vi "climb mode.vi"(4 "i":i32=1508, 6 "Joystick 2":T1, 7 "Arm Angle":dbl=0.38043151000000003, 8 "engage climb":bool, 9 "Button 1":bool, 10 "Slide":dbl(slide)=1.0 scale=0.0..1.0, 11 "Joystick 1 Axes":T2={"Axis 1 (x)"=0.047244094488188976, "Axis 2 (y)"=-0.047244094488188976, "Axis 3 (throttle)"=-1.0, "Axis 4"=0.0, "Axis 5"=0.0, "Axis 6"=0.0}) -> ()   [LabVIEW 2012]
uses:
  <vilib>/Rock Robotics/WPI/Solenoid/WPI_SolenoidValue.ctl
  <vilib>/Rock Robotics/WPI/Joystick/WPI_JoystickGetSetRefNum.vi
  <vilib>/Rock Robotics/WPI/Solenoid/WPI_SolenoidSetEnum.vi
panel:
  out "Arm Motor Output":dbl
  out "Down Range":dbl=0.6
  out "Up Range":dbl=4.1
  out "right f":i32=11868
  out "left f":i32=11868
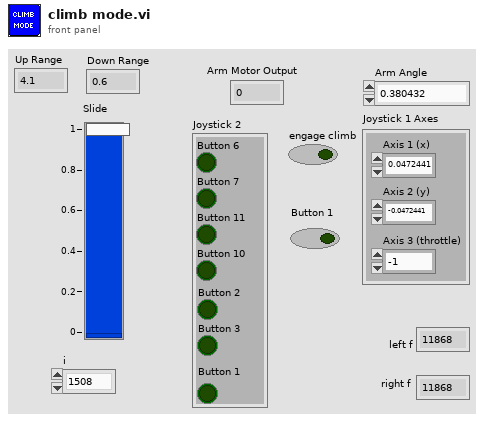
[diagram p1: front panel]
types:
  T1 = cluster{"Button 6":bool, "Button 7":bool, "Button 11":bool, "Button 10":bool, "Button 2":bool, "Button 3":bool, "Button 1":bool}
  T2 = cluster{"Axis 1 (x)":dbl, "Axis 2 (y)":dbl, "Axis 3 (throttle)":dbl, "Axis 4":dbl, "Axis 5":dbl, "Axis 6":dbl}
  T3 = typedef "WPI_SolenoidValue.ctl" = enum16{"Off", "On", "Forward", "Reverse"}
  T4 = typedef "WPI_JoystickDevRef.ctl" = cluster{"Device":T5}
  T5 = typedef "WPI_JoystickDeviceEnum.ctl" = enum16{"USB 1", "USB 2", "USB 3", "USB 4", "Kinect 1", "Kinect 2"}
  T6 = typedef "WPI_JoystickButtonState.ctl" = cluster{"Button 1":bool, "Button 2":bool, "Button 3":bool, "Button 4":bool, "Button 5":bool, "Button 6":bool, "Button 7":bool, "Button 8":bool, "Button 9":bool, "Button 10":bool, "Button 11":bool, "Button 12":bool}
  T7 = typedef "WPI_SolenoidDevRef.ctl" = cluster{"DevStatus":errorcluster, "Solenoid Module":T8, "Forward Solenoid Channel":T9, "Reverse Solenoid Channel":T9}
  T8 = typedef "FPGA_TypedefSolenoidModule.ctl" = enum16{"Solenoid Module 1", "Solenoid Module 2"}
  T9 = typedef "WPI_SolenoidChannel.ctl" = enum8{"Solenoid 1", "Solenoid 2", "Solenoid 3", "Solenoid 4", "Solenoid 5", "Solenoid 6", "Solenoid 7", "Solenoid 8", "Invalid"}
  T10 = typedef "WPI_MotorControlDeviceRef.ctl" = cluster{"DeviceStatus":errorcluster, "Type":enum16{"PWM", "CAN"}, "PWM":cluster{"Digital Module":T11, "PWM Channel":T12, "DeadBand":T13}, "CAN":cluster{"Device Number":u8, "Control Mode":T14, "Semaphore":T15, "Max Vout":dbl}, "Invert":bool, "TransformRef":T16, "InvTransformRef":T16}
  T11 = typedef "FPGA_TypedefDigitalModule.ctl" = enum16{"Digital Module 1", "Digital Module 2"}
  T12 = typedef "FPGA_DIOPWMChannel.ctl" = enum8{"PWM 1", "PWM 2", "PWM 3", "PWM 4", "PWM 5", "PWM 6", "PWM 7", "PWM 8", "PWM 9", "PWM 10", "Invalid"}
  T13 = typedef "WPI_PWMDeadband.ctl" = cluster{"Name":string, "maxPositivePwm":i32, "minPositivePwm":i32, "centerPwm":i32, "maxNegativePwm":i32, "minNegativePwm":i32, "angularRange":u16}
  T14 = typedef "WPI_CANJaguar_ControlMode.ctl" = enum8{"Percent VBus", "Current", "Speed", "Position", "Voltage"}
  T15 = typedef "Semaphore RefNum" = refnum<k1>
  T16 = typedef "WPI_PWMTransform_ConPane.ctl" = refnum<vi>
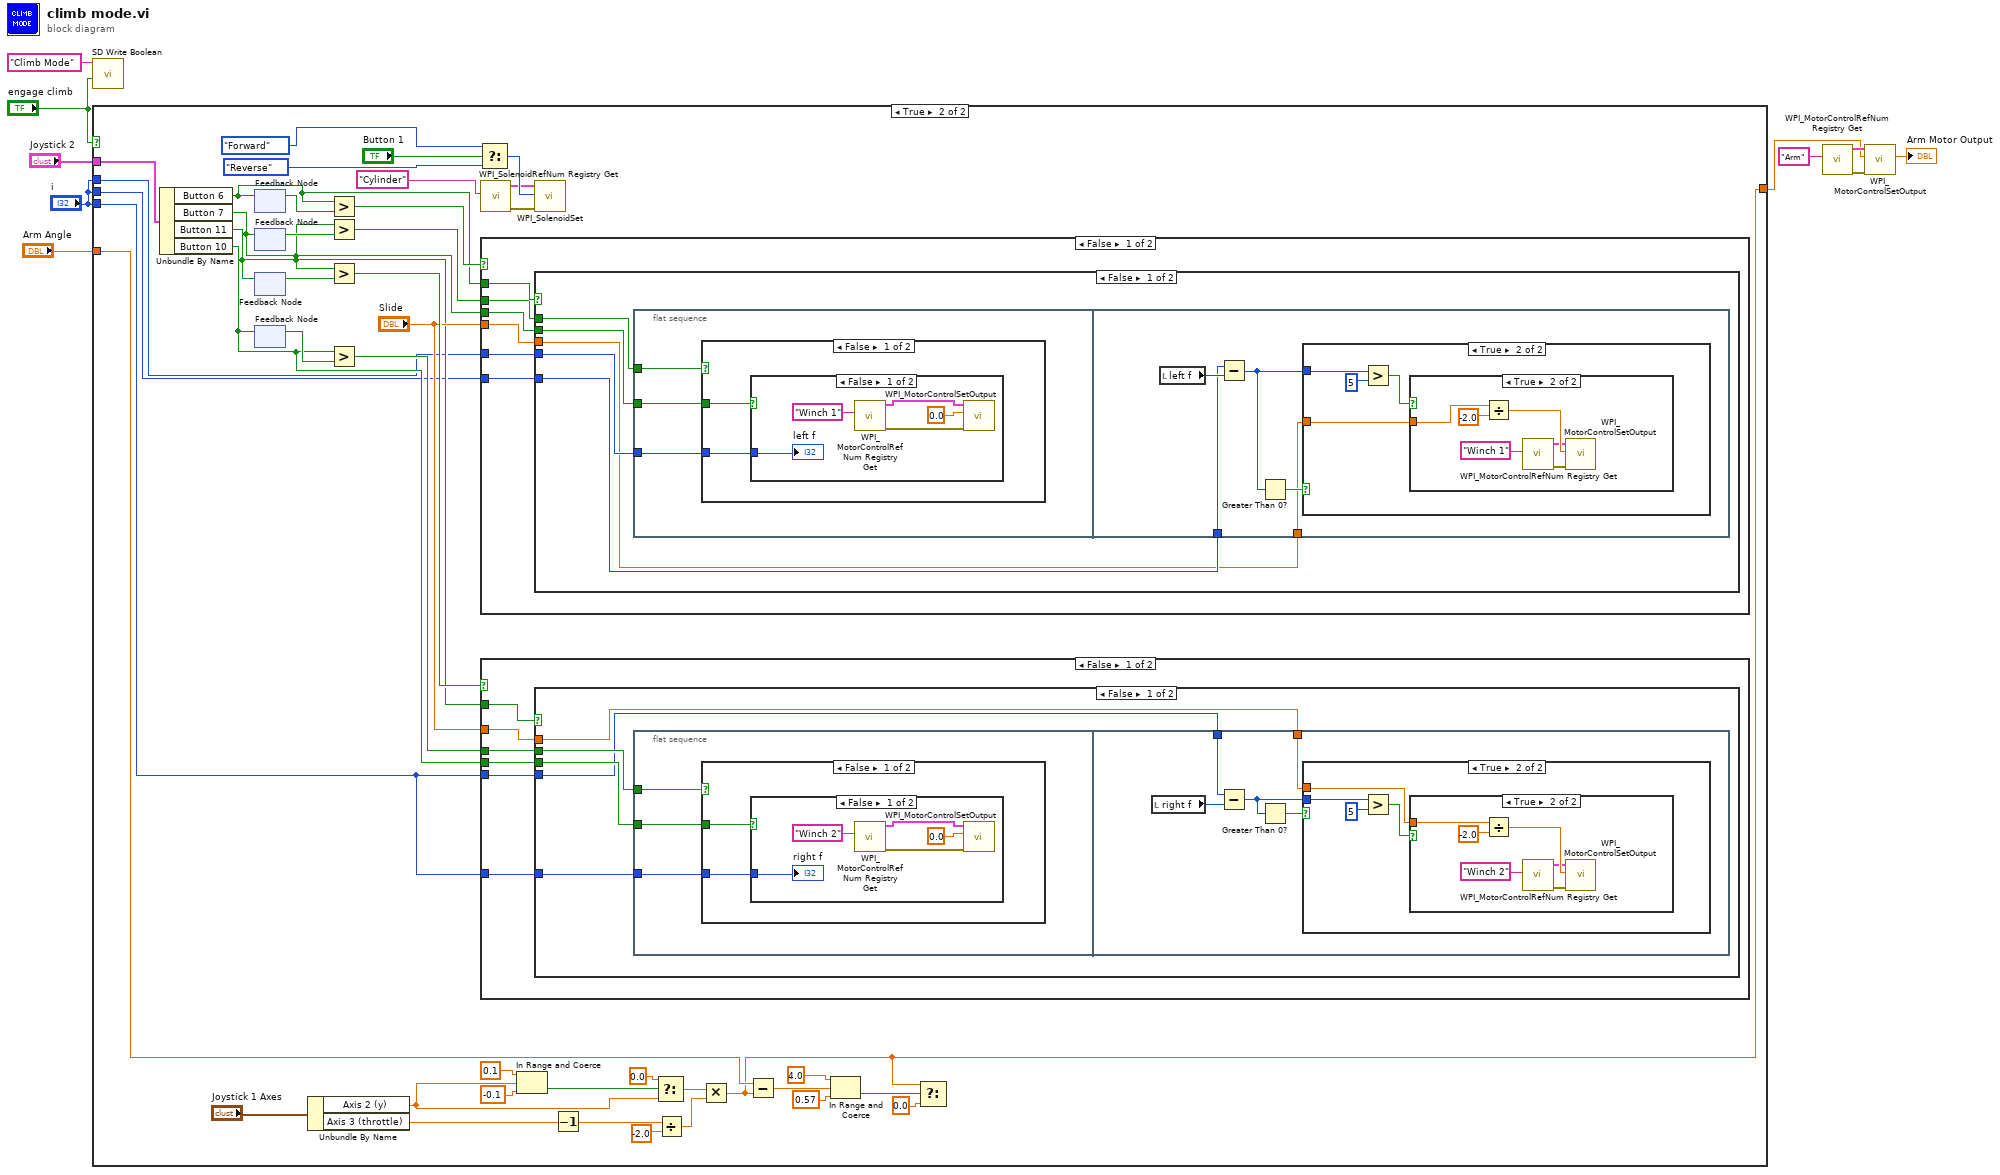
[diagram p0: block diagram]
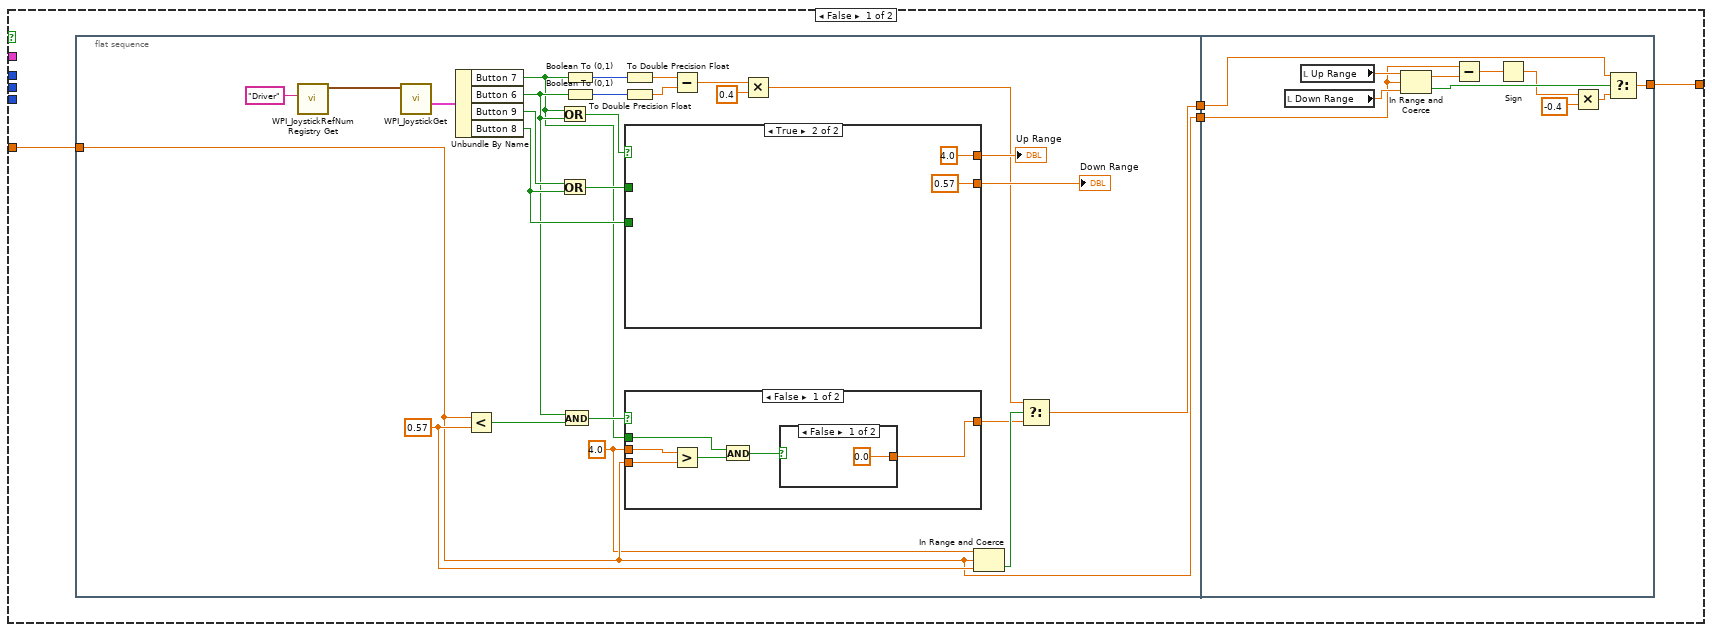
[diagram p2: hidden frame]
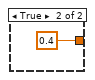
[diagram p3: hidden frame]
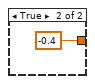
[diagram p4: hidden frame]
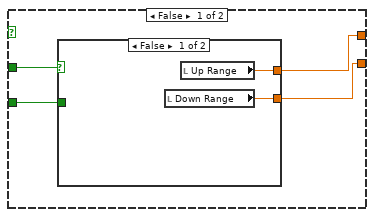
[diagram p5: hidden frame]
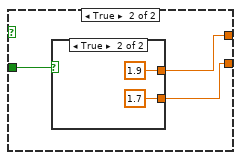
[diagram p6: hidden frame]
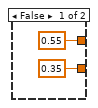
[diagram p7: hidden frame]
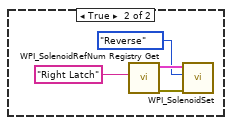
[diagram p8: hidden frame]
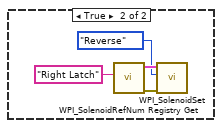
[diagram p9: hidden frame]
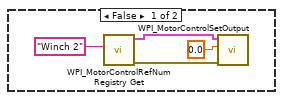
[diagram p10: hidden frame]
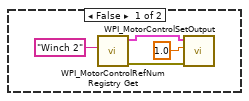
[diagram p11: hidden frame]
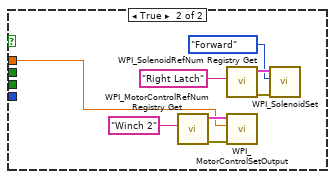
[diagram p12: hidden frame]
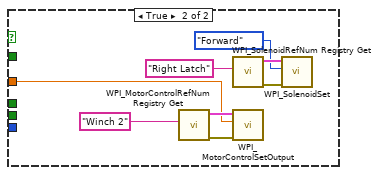
[diagram p13: hidden frame]
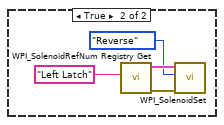
[diagram p14: hidden frame]
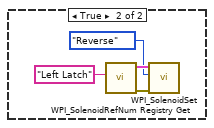
[diagram p15: hidden frame]
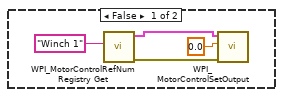
[diagram p16: hidden frame]
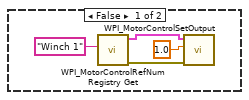
[diagram p17: hidden frame]
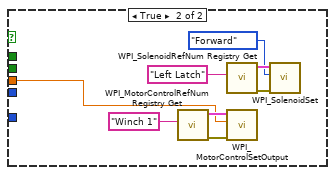
[diagram p18: hidden frame]
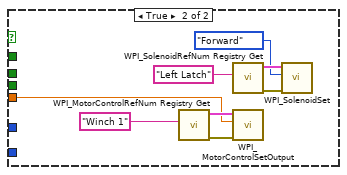
[diagram p19: hidden frame]
diagram:
  n1 = call <vilib>:"SD Write Boolean.vi"("Boolean"="engage climb", "Name"="Climb Mode") -> ()  [unwired: 8 in, 2 out]
  n2 = case shown="True" "engage climb" {
    tunnel: "Joystick 2" -> [_ w109]
    tunnel: "i" -> [_ w95]
    tunnel: "i" -> [_ w94]
    tunnel: "i" -> [_ w93]
    tunnel: "Arm Angle" -> [w14 w87]
    tunnel: [w11 w82] -> w2
    frame False {
      n3 = flat-sequence {
        tunnel: w14 -> [w16]
        tunnel: [w23] -> w13
        tunnel: [w16] -> w12
        tunnel: w13 -> [w66]
        tunnel: w12 -> [w71]
        tunnel: [w65] -> w11
        frame #0 {
          w22 = 0.57 ("lower limit")
          w15 = 4.0 ("upper limit")
          n4 = call <vilib>:"WPI_JoystickRefNum Registry Get.vi"("refnum name"="Driver") -> ("JoystickDevRef"=w40:T4)  [unwired: 9 in, 1 out]
          n5 = call <vilib>:"WPI_JoystickGet.vi"("JoystickDevRef"=w40) -> ("Buttons"=w38:T6)  [unwired: 4 in, 2 out]
          n6 = Unbundle By Name(w38) -> ("Button 7"=w17:bool, "Button 6"=w18:bool, "Button 9"=w29:bool, "Button 8"=w25:bool)
          n7 = Less?(x=w16, y=w22) -> (x < y?=w20:bool)
          n8 = Or(x=w17, y=w18) -> (x .or. y?=w28:bool)
          n9 = Or(x=w29, y=w25) -> (x .or. y?=w30:bool)
          n10 = And(x=w18, y=w20) -> (x .and. y?=w19:bool)
          n11 = Boolean To (0,1)(Boolean=w17) -> (0, 1=w37:i16)
          n12 = Boolean To (0,1)(Boolean=w18) -> (0, 1=w36:i16)
          n13 = To Double Precision Float(number=w37) -> (double precision float=w35:dbl)
          n14 = To Double Precision Float(number=w36) -> (double precision float=w34:dbl)
          n15 = case shown="True" w28 {
            tunnel: w30 -> [w53 _]
            tunnel: [w52 4.0] -> w27
            tunnel: [w51 0.57] -> w26
            tunnel: w25 -> [w50 _]
            frame False {
              n16 = case shown="False" w53 {
                tunnel: [w55 w56] -> w52
                tunnel: [w54 w57] -> w51
                tunnel: w50 -> [_ w58]
                frame False {
                  n17 = local read "Down Range"() -> (w54:dbl)
                  n18 = local read "Up Range"() -> (w55:dbl)
                }
                frame True {
                  n19 = case shown="True" w58 {
                    tunnel: [0.35 1.7] -> w57
                    tunnel: [0.55 1.9] -> w56
                    frame False {
                    }
                    frame True {
                    }
                  }
                }
              }
            }
            frame True {
            }
          }
          "Up Range" <- w27
          "Down Range" <- w26
          n20 = case shown="False" w19 {
            tunnel: [w41 -0.4 ("t")] -> w21
            tunnel: w17 -> [w45 _]
            tunnel: w16 -> [w43 _]
            tunnel: w15 -> [w42 _]
            frame False {
              n21 = Greater?(x=w42, y=w43) -> (0:w44:bool)
              n22 = And(x=w45, y=w44) -> (x .and. y?=w46:bool)
              n23 = case shown="False" w46 {
                tunnel: [0.0 0.4] -> w41
                frame False {
                }
                frame True {
                }
              }
            }
            frame True {
            }
          }
          n24 = Subtract(x=w35, y=w34) -> (x-y=w32:dbl)
          n25 = Multiply(x=w32, y=0.4) -> (x*y=w24:dbl)
          n26 = In Range and Coerce(upper limit=w15, x=w16, lower limit=w22) -> (In Range?=w31:bool)  [unwired: 1 out]
          n27 = Select(t=w24, s=w31, f=w21) -> (s? t:f=w23:dbl)
        }
        frame #1 {
          n28 = local read "Down Range"() -> (w75:dbl)
          n29 = local read "Up Range"() -> (w74:dbl)
          n30 = In Range and Coerce(upper limit=w74, x=w71, lower limit=w75) -> (coerced(x)=w72:dbl, In Range?=w73:bool)
          n31 = Subtract(x=w71, y=w72) -> (x-y=w70:dbl)
          n32 = Sign(1:w70) -> (0:w69:dbl)
          n33 = Multiply(x=w69, y=-0.4) -> (x*y=w67:dbl)
          n34 = Select(t=w66, s=w73, f=w67) -> (s? t:f=w65:dbl)
        }
      }
    }
    frame True {
      n35 = Unbundle By Name(w109) -> ("Button 6"=w99:bool, "Button 7"=w98:bool, "Button 11"=w97:bool, "Button 10"=w96:bool)
      n36 = feedback-in #1(w99) -> ()
      n37 = feedback #1() -> (w108:bool)  [unwired: 1 in]
      n38 = feedback #2() -> (w107:bool)  [unwired: 1 in]
      n39 = feedback-in #2(w98) -> ()
      n40 = feedback #3() -> (w104:bool)  [unwired: 1 in]
      n41 = feedback-in #3(w97) -> ()
      n42 = feedback #4() -> (w103:bool)  [unwired: 1 in]
      n43 = feedback-in #4(w96) -> ()
      n44 = Unbundle By Name("Joystick 1 Axes") -> ("Axis 2 (y)"=w77:dbl, "Axis 3 (throttle)"=w86:dbl)
      n45 = Greater?(x=w99, y=w108) -> (0:w106:bool)
      n46 = Greater?(x=w98, y=w107) -> (0:w105:bool)
      n47 = Greater?(x=w97, y=w104) -> (0:w102:bool)
      n48 = Greater?(x=w96, y=w103) -> (0:w101:bool)
      n49 = Select(t=WPI_SolenoidValue."Forward", s="Button 1", f=WPI_SolenoidValue."Reverse" ("Value")) -> (s? t:f=w114:T3)
      n50 = call <vilib>:"WPI_SolenoidRefNum Registry Get.vi"("refnum name"="Cylinder") -> ("error out"=w110:errorcluster, "SolenoidDevRef"=w113:T7)  [unwired: 9 in]
      n51 = case shown="False" w106 {
        tunnel: "Slide" -> [w190 w246]
        tunnel: w99 -> [w191 _]
        tunnel: w105 -> [w189 _]
        tunnel: w98 -> [w188 _]
        tunnel: w95 -> [w187 _]
        tunnel: w94 -> [w186 _]
        frame False {
          n52 = case shown="False" w191 {
            tunnel: w190 -> [w192 w242]
            tunnel: w188 -> [w196 _]
            tunnel: w189 -> [w195 _]
            tunnel: w187 -> [w194 _]
            tunnel: w186 -> [w193 _]
            frame False {
              n53 = flat-sequence {
                tunnel: w196 -> [w199]
                tunnel: w195 -> [w198]
                tunnel: w194 -> [w197]
                tunnel: w193 -> [w216]
                tunnel: w192 -> [w215]
                frame #0 {
                  n54 = case shown="False" w198 {
                    tunnel: w199 -> [w201 _]
                    tunnel: w197 -> [w200 _]
                    frame False {
                      n55 = case shown="False" w201 {
                        tunnel: w200 -> [w206 _]
                        frame False {
                          n56 = call <vilib>:"WPI_MotorControlRefNum Registry Get.vi"("refnum name"="Winch 1") -> ("error out"=w205:errorcluster, "MotorControlDevRef"=w203:T10)  [unwired: 9 in]
                          n57 = call <vilib>:"WPI_MotorControlSetOutput.vi"("error in (no error)"=w205, "Output"=0.0, "MotorControlDevRef"=w203) -> ()  [unwired: 6 in, 3 out]
                          "left f" <- w206
                        }
                        frame True {
                          n58 = call <vilib>:"WPI_SolenoidRefNum Registry Get.vi"("refnum name"="Left Latch") -> ("error out"=w210:errorcluster, "SolenoidDevRef"=w208:T7)  [unwired: 9 in]
                          n59 = call-poly <vilib>:"WPI_SolenoidSet.vi"("error in (no error)"=w210, "Value"=WPI_SolenoidValue."Reverse", "SolenoidDevRef"=w208) -> ()  [unwired: 7 in, 2 out]
                        }
                      }
                    }
                    frame True {
                      n60 = call <vilib>:"WPI_SolenoidRefNum Registry Get.vi"("refnum name"="Left Latch") -> ("error out"=w214:errorcluster, "SolenoidDevRef"=w212:T7)  [unwired: 9 in]
                      n61 = call-poly <vilib>:"WPI_SolenoidSet.vi"("error in (no error)"=w214, "Value"=WPI_SolenoidValue."Reverse", "SolenoidDevRef"=w212) -> ()  [unwired: 7 in, 2 out]
                    }
                  }
                }
                frame #1 {
                  n62 = local read "left f"() -> (w218:i32)
                  n63 = Subtract(x=w216, y=w218) -> (x-y=w219:i32)
                  n64 = Greater Than 0?(x=w219) -> (x > 0?=w217:bool)
                  n65 = case shown="True" w217 {
                    tunnel: w219 -> [_ w225]
                    tunnel: w215 -> [_ w224]
                    frame False {
                      n66 = call <vilib>:"WPI_MotorControlRefNum Registry Get.vi"("refnum name"="Winch 1") -> ("error out"=w223:errorcluster, "MotorControlDevRef"=w221:T10)  [unwired: 9 in]
                      n67 = call <vilib>:"WPI_MotorControlSetOutput.vi"("error in (no error)"=w223, "Output"=0.0, "MotorControlDevRef"=w221) -> ()  [unwired: 6 in, 3 out]
                    }
                    frame True {
                      n68 = Greater?(x=w225, y=5) -> (0:w227:bool)
                      n69 = case shown="True" w227 {
                        tunnel: w224 -> [_ w232]
                        frame False {
                          n70 = call <vilib>:"WPI_MotorControlRefNum Registry Get.vi"("refnum name"="Winch 1") -> ("error out"=w231:errorcluster, "MotorControlDevRef"=w229:T10)  [unwired: 9 in]
                          n71 = call <vilib>:"WPI_MotorControlSetOutput.vi"("error in (no error)"=w231, "Output"=1.0, "MotorControlDevRef"=w229) -> ()  [unwired: 6 in, 3 out]
                        }
                        frame True {
                          n72 = Divide(x=w232, y=-2.0) -> (x/y=w237:dbl)
                          n73 = call <vilib>:"WPI_MotorControlRefNum Registry Get.vi"("refnum name"="Winch 1") -> ("error out"=w236:errorcluster, "MotorControlDevRef"=w234:T10)  [unwired: 9 in]
                          n74 = call <vilib>:"WPI_MotorControlSetOutput.vi"("error in (no error)"=w236, "Output"=w237, "MotorControlDevRef"=w234) -> ()  [unwired: 6 in, 3 out]
                        }
                      }
                    }
                  }
                }
              }
            }
            frame True {
              n75 = call <vilib>:"WPI_MotorControlRefNum Registry Get.vi"("refnum name"="Winch 1") -> ("error out"=w245:errorcluster, "MotorControlDevRef"=w243:T10)  [unwired: 9 in]
              n76 = call <vilib>:"WPI_SolenoidRefNum Registry Get.vi"("refnum name"="Left Latch") -> ("error out"=w241:errorcluster, "SolenoidDevRef"=w239:T7)  [unwired: 9 in]
              n77 = call <vilib>:"WPI_MotorControlSetOutput.vi"("error in (no error)"=w245, "Output"=w242, "MotorControlDevRef"=w243) -> ()  [unwired: 6 in, 3 out]
              n78 = call-poly <vilib>:"WPI_SolenoidSet.vi"("error in (no error)"=w241, "Value"=WPI_SolenoidValue."Forward", "SolenoidDevRef"=w239) -> ()  [unwired: 7 in, 2 out]
            }
          }
        }
        frame True {
          n79 = call <vilib>:"WPI_MotorControlRefNum Registry Get.vi"("refnum name"="Winch 1") -> ("error out"=w249:errorcluster, "MotorControlDevRef"=w247:T10)  [unwired: 9 in]
          n80 = call <vilib>:"WPI_SolenoidRefNum Registry Get.vi"("refnum name"="Left Latch") -> ("error out"=w253:errorcluster, "SolenoidDevRef"=w251:T7)  [unwired: 9 in]
          n81 = call <vilib>:"WPI_MotorControlSetOutput.vi"("error in (no error)"=w249, "Output"=w246, "MotorControlDevRef"=w247) -> ()  [unwired: 6 in, 3 out]
          n82 = call-poly <vilib>:"WPI_SolenoidSet.vi"("error in (no error)"=w253, "Value"=WPI_SolenoidValue."Forward", "SolenoidDevRef"=w251) -> ()  [unwired: 7 in, 2 out]
        }
      }
      n83 = case shown="False" w102 {
        tunnel: "Slide" -> [w122 w178]
        tunnel: w97 -> [w123 _]
        tunnel: w101 -> [w121 _]
        tunnel: w96 -> [w120 _]
        tunnel: w93 -> [w119 _]
        tunnel: w93 -> [w118 _]
        frame False {
          n84 = case shown="False" w123 {
            tunnel: w122 -> [w124 w174]
            tunnel: w120 -> [w128 _]
            tunnel: w121 -> [w127 _]
            tunnel: w119 -> [w125 _]
            tunnel: w118 -> [w126 _]
            frame False {
              n85 = flat-sequence {
                tunnel: w128 -> [w131]
                tunnel: w127 -> [w130]
                tunnel: w126 -> [w129]
                tunnel: w125 -> [w148]
                tunnel: w124 -> [w147]
                frame #0 {
                  n86 = case shown="False" w130 {
                    tunnel: w131 -> [w133 _]
                    tunnel: w129 -> [w132 _]
                    frame False {
                      n87 = case shown="False" w133 {
                        tunnel: w132 -> [w138 _]
                        frame False {
                          n88 = call <vilib>:"WPI_MotorControlRefNum Registry Get.vi"("refnum name"="Winch 2") -> ("error out"=w137:errorcluster, "MotorControlDevRef"=w135:T10)  [unwired: 9 in]
                          n89 = call <vilib>:"WPI_MotorControlSetOutput.vi"("error in (no error)"=w137, "Output"=0.0, "MotorControlDevRef"=w135) -> ()  [unwired: 6 in, 3 out]
                          "right f" <- w138
                        }
                        frame True {
                          n90 = call <vilib>:"WPI_SolenoidRefNum Registry Get.vi"("refnum name"="Right Latch") -> ("error out"=w142:errorcluster, "SolenoidDevRef"=w140:T7)  [unwired: 9 in]
                          n91 = call-poly <vilib>:"WPI_SolenoidSet.vi"("error in (no error)"=w142, "Value"=WPI_SolenoidValue."Reverse", "SolenoidDevRef"=w140) -> ()  [unwired: 7 in, 2 out]
                        }
                      }
                    }
                    frame True {
                      n92 = call <vilib>:"WPI_SolenoidRefNum Registry Get.vi"("refnum name"="Right Latch") -> ("error out"=w146:errorcluster, "SolenoidDevRef"=w144:T7)  [unwired: 9 in]
                      n93 = call-poly <vilib>:"WPI_SolenoidSet.vi"("error in (no error)"=w146, "Value"=WPI_SolenoidValue."Reverse", "SolenoidDevRef"=w144) -> ()  [unwired: 7 in, 2 out]
                    }
                  }
                }
                frame #1 {
                  n94 = local read "right f"() -> (w150:i32)
                  n95 = Subtract(x=w148, y=w150) -> (x-y=w151:i32)
                  n96 = Greater Than 0?(x=w151) -> (x > 0?=w149:bool)
                  n97 = case shown="True" w149 {
                    tunnel: w151 -> [_ w157]
                    tunnel: w147 -> [_ w156]
                    frame False {
                      n98 = call <vilib>:"WPI_MotorControlRefNum Registry Get.vi"("refnum name"="Winch 2") -> ("error out"=w155:errorcluster, "MotorControlDevRef"=w153:T10)  [unwired: 9 in]
                      n99 = call <vilib>:"WPI_MotorControlSetOutput.vi"("error in (no error)"=w155, "Output"=0.0, "MotorControlDevRef"=w153) -> ()  [unwired: 6 in, 3 out]
                    }
                    frame True {
                      n100 = Greater?(x=w157, y=5) -> (0:w159:bool)
                      n101 = case shown="True" w159 {
                        tunnel: w156 -> [_ w164]
                        frame False {
                          n102 = call <vilib>:"WPI_MotorControlRefNum Registry Get.vi"("refnum name"="Winch 2") -> ("error out"=w163:errorcluster, "MotorControlDevRef"=w161:T10)  [unwired: 9 in]
                          n103 = call <vilib>:"WPI_MotorControlSetOutput.vi"("error in (no error)"=w163, "Output"=1.0, "MotorControlDevRef"=w161) -> ()  [unwired: 6 in, 3 out]
                        }
                        frame True {
                          n104 = Divide(x=w164, y=-2.0) -> (x/y=w169:dbl)
                          n105 = call <vilib>:"WPI_MotorControlRefNum Registry Get.vi"("refnum name"="Winch 2") -> ("error out"=w168:errorcluster, "MotorControlDevRef"=w166:T10)  [unwired: 9 in]
                          n106 = call <vilib>:"WPI_MotorControlSetOutput.vi"("error in (no error)"=w168, "Output"=w169, "MotorControlDevRef"=w166) -> ()  [unwired: 6 in, 3 out]
                        }
                      }
                    }
                  }
                }
              }
            }
            frame True {
              n107 = call <vilib>:"WPI_MotorControlRefNum Registry Get.vi"("refnum name"="Winch 2") -> ("error out"=w177:errorcluster, "MotorControlDevRef"=w175:T10)  [unwired: 9 in]
              n108 = call <vilib>:"WPI_SolenoidRefNum Registry Get.vi"("refnum name"="Right Latch") -> ("error out"=w173:errorcluster, "SolenoidDevRef"=w171:T7)  [unwired: 9 in]
              n109 = call <vilib>:"WPI_MotorControlSetOutput.vi"("error in (no error)"=w177, "Output"=w174, "MotorControlDevRef"=w175) -> ()  [unwired: 6 in, 3 out]
              n110 = call-poly <vilib>:"WPI_SolenoidSet.vi"("error in (no error)"=w173, "Value"=WPI_SolenoidValue."Forward", "SolenoidDevRef"=w171) -> ()  [unwired: 7 in, 2 out]
            }
          }
        }
        frame True {
          n111 = call <vilib>:"WPI_MotorControlRefNum Registry Get.vi"("refnum name"="Winch 2") -> ("error out"=w181:errorcluster, "MotorControlDevRef"=w179:T10)  [unwired: 9 in]
          n112 = call <vilib>:"WPI_SolenoidRefNum Registry Get.vi"("refnum name"="Right Latch") -> ("error out"=w185:errorcluster, "SolenoidDevRef"=w183:T7)  [unwired: 9 in]
          n113 = call <vilib>:"WPI_MotorControlSetOutput.vi"("error in (no error)"=w181, "Output"=w178, "MotorControlDevRef"=w179) -> ()  [unwired: 6 in, 3 out]
          n114 = call-poly <vilib>:"WPI_SolenoidSet.vi"("error in (no error)"=w185, "Value"=WPI_SolenoidValue."Forward", "SolenoidDevRef"=w183) -> ()  [unwired: 7 in, 2 out]
        }
      }
      n115 = In Range and Coerce(upper limit=0.1, x=w77, lower limit=-0.1) -> (In Range?=w79:bool)  [unwired: 1 out]
      n116 = call-poly <vilib>:"WPI_SolenoidSet.vi"("error in (no error)"=w110, "Value"=w114, "SolenoidDevRef"=w113) -> ()  [unwired: 7 in, 2 out]
      n117 = Decrement(x=w86) -> (x-1=w85:dbl)
      n118 = Select(t=0.0, s=w79, f=w77) -> (s? t:f=w76:dbl)
      n119 = Divide(x=w85, y=-2.0) -> (x/y=w83:dbl)
      n120 = Multiply(x=w76, y=w83) -> (x*y=w82:dbl)
      n121 = Subtract(x=w87, y=w82) -> (x-y=w90:dbl)
      n122 = In Range and Coerce(upper limit=4.0, x=w90, lower limit=0.57) -> (In Range?=w91:bool)  [unwired: 1 out]
      n123 = Select(t=w82, s=w91, f=0.0) -> ()  [unwired: 1 out]
    }
  }
  n124 = call <vilib>:"WPI_MotorControlRefNum Registry Get.vi"("refnum name"="Arm") -> ("error out"=w4:errorcluster, "MotorControlDevRef"=w3:T10)  [unwired: 9 in]
  n125 = call <vilib>:"WPI_MotorControlSetOutput.vi"("error in (no error)"=w4, "Output"=w2, "MotorControlDevRef"=w3) -> ("Motor Output"=→"Arm Motor Output":dbl)  [unwired: 6 in, 2 out]
